vi "PDCUpdateFrameNo.vi"(8 "Error In":errorcluster, 10 "PDCAllStates in":T1={"DeviceNo"=0, "ChildNo"=1, "ColorType"=enum."MONO", "BitDepth"=0, "Resolution"={"Width"=0, "Height"=0}, "RecordRate"=0, "ShutterSpeed"=0, "TriggerMode"=0, "Display"=enum."LiveStop", "PDCRecordStatus"=enum."Live", "PlayFrames"=FALSE, "Start Frame"=0, "Current Frame"=0, "End Frame"=0, "RefImage8bit"=[], "RefImage16bit"=[], "Auto Trigger"=FALSE, "PDCSettings"={"Interface"=enum."Gigabit-Ethernet", "AutoSearch"=FALSE, "IP - AutoSearch"=[], "IP - Direct"=[], "Simulate"=FALSE}}, 11 "DataDisplayQueue":refnum<queue>) -> (0 "Error Out":errorcluster, 2 "PDCAllStates out":T1={"DeviceNo"=0, "ChildNo"=1, "ColorType"=enum."MONO", "BitDepth"=0, "Resolution"={"Width"=0, "Height"=0}, "RecordRate"=0, "ShutterSpeed"=0, "TriggerMode"=0, "Display"=enum."LiveStop", "PDCRecordStatus"=enum."Live", "PlayFrames"=FALSE, "Start Frame"=0, "Current Frame"=0, "End Frame"=0, "RefImage8bit"=[], "RefImage16bit"=[], "Auto Trigger"=FALSE, "PDCSettings"={"Interface"=enum."Gigabit-Ethernet", "AutoSearch"=FALSE, "IP - AutoSearch"=[], "IP - Direct"=[], "Simulate"=FALSE}})   [LabVIEW 2015]
uses:
  TypeDefs/PDCAllStates.ctl
  TypeDefs/PDCDisplay.ctl
  TypeDefs/PDCRecordStatus.ctl
  TypeDefs/PDCSettings.ctl
  TypeDefs/MessageCluster.ctl
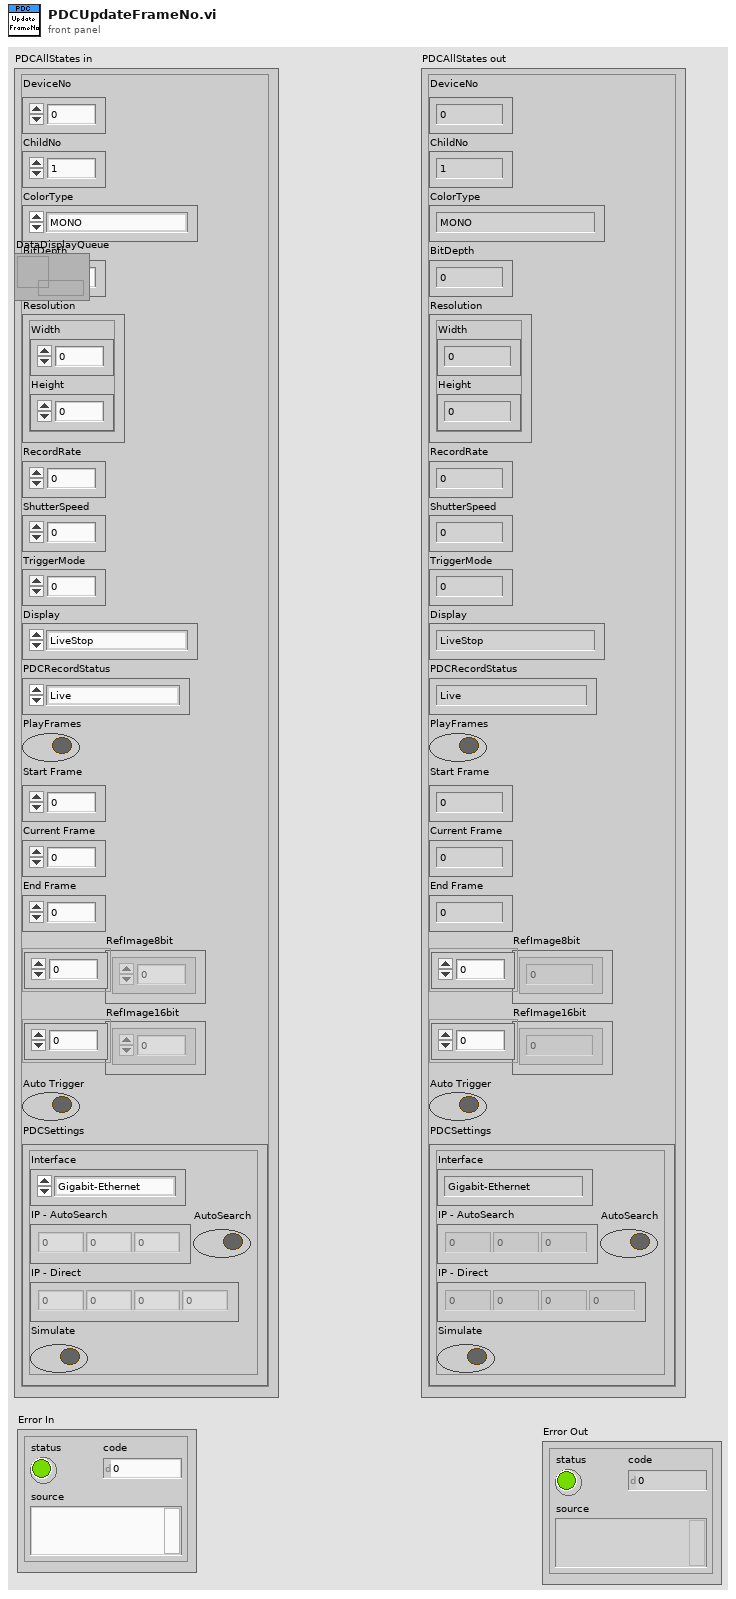
[diagram p1: front panel]
types:
  T1 = typedef "PDCAllStates.ctl" = cluster{"DeviceNo":u32, "ChildNo":u32, "ColorType":enum16{"MONO", "COLOR"}, "BitDepth":i8, "Resolution":cluster{"Width":u32, "Height":u32}, "RecordRate":u32, "ShutterSpeed":u32, "TriggerMode":u32, "Display":T2, "PDCRecordStatus":T3, "PlayFrames":bool, "Start Frame":i32, "Current Frame":i32, "End Frame":i32, "RefImage8bit":u8[], "RefImage16bit":u16[], "Auto Trigger":bool, "PDCSettings":T4}
  T2 = typedef "PDCDisplay.ctl" = enum16{"Live", "Memory", "LiveStop"}
  T3 = typedef "PDCRecordStatus.ctl" = enum16{"Live", "Waiting TRG", "Recording"}
  T4 = typedef "PDCSettings.ctl" = cluster{"Interface":enum16{"Gigabit-Ethernet", "IEEE1394a", "Photron Optical", "PCI/PCI Express"}, "AutoSearch":bool, "IP - AutoSearch":u32[], "IP - Direct":u32[], "Simulate":bool}
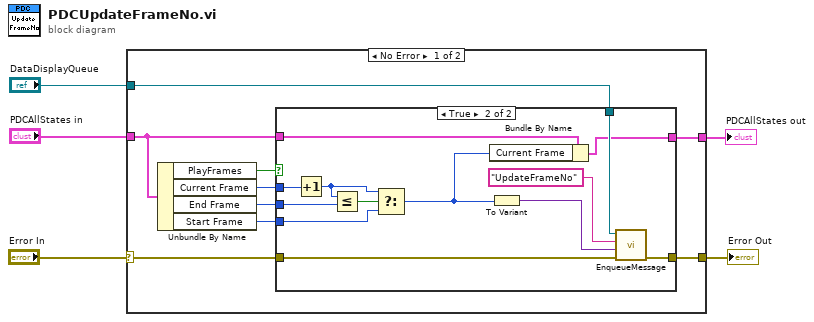
[diagram p0: block diagram]
diagram:
  n1 = case shown="No Error" "Error In" {
    selector: "Error In" -> [w14 w31]
    tunnel: "DataDisplayQueue" -> [w12 _]
    tunnel: [w13 w31] -> w3
    tunnel: "PDCAllStates in" -> [w7 w30]
    tunnel: [w6 w30] -> w1
    frame No Error {
      n2 = Unbundle By Name(w7) -> ("PlayFrames"=w11:bool, "Current Frame"=w10:i32, "End Frame"=w9:i32, "Start Frame"=w8:i32)
      n3 = case shown="True" w11 {
        tunnel: w14 -> [w16 w29]
        tunnel: [w16 w28] -> w13
        tunnel: w12 -> [_ w27]
        tunnel: w10 -> [_ w26]
        tunnel: w9 -> [_ w25]
        tunnel: w8 -> [_ w22]
        tunnel: w7 -> [w15 w19]
        tunnel: [w15 w17] -> w6
        frame False {
        }
        frame True {
          n4 = Increment(x=w26) -> (x+1=w23:i32)
          n5 = Less Or Equal?(x=w23, y=w25) -> (x <= y?=w24:bool)
          n6 = Select(t=w23, s=w24, f=w22) -> (s? t:f=w18:i32)
          n7 = Bundle By Name(cluster=w19, "Current Frame"=w18) -> (w17:T1)
          n8 = To Variant(anything=w18) -> (Variant=w21:variant)
          n9 = call "EnqueueMessage.vi"("error in (no error)"=w29, "MessageData"=w21, "Message"="UpdateFrameNo", "MessageQueue"=w27) -> ("error out"=w28:errorcluster)  [unwired: 6 in, 1 out]
        }
      }
    }
    frame Error {
    }
  }
  "Error Out" <- w3
  "PDCAllStates out" <- w1
